vi "FPGA_VI.vi"() -> ()   [LabVIEW 2014]
uses:
  FPGA_Controls/IOClockState.ctl
  <vilib>/Platform/TimedLoop/XDataNode/timing_clust.ctl
  <vilib>/Platform/TimedLoop/XDataNode/nitl_modes.ctl
  <vilib>/Platform/TimedLoop/XDataNode/wakeup.ctl
  FPGA_Controls/DRAMClockState.ctl
  <vilib>/rvi/Emulation/niFpgaSctlEmulationGetInTimedLoop.vi
  <vilib>/rvi/Emulation/niFpgaEmulationReportErrorSimple.vi
  <vilib>/rvi/Emulation/niFpgaGetClockAttributes.vi
  <vilib>/rvi/Emulation/niFpgaCriticalErrorInLSC.vi
  <vilib>/rvi/eio/common/nirviEmuTemplateMethod_errors.vi
  <vilib>/rvi/Emulation/niFpgaEmulationIsFPGAContextNoSignature.vi
  <vilib>/rvi/errors/niFpgaSetErrorForExecOnDevCompSimple.vi
  <vilib>/rvi/eio/common/nirviEmuReportErrorAndStop.vi
  <vilib>/rvi/DataTransferAndStorage/Container/Common/niFpgaContainerGetUniqueNameForEmu.vi
  <vilib>/rvi/FIFO/Fifo_Resource/nirvififoEmulationSetSize.vi
  <vilib>/rvi/FIFO/Fifo_Resource/nirviFifoEmulationQueueMgr.vi
  <instcachedir>/0/nirviFifoEmulationQueueMgr_E5CAEC123FF24DC58D834DCA3CDAA9B5.lvgen/nirviFifoEmulationQueueMgr_E5CAEC123FF24DC58D834DCA3CDAA9B5_002.vi
  <vilib>/Utility/error.llb/Clear Errors.vi
  <vilib>/rvi/FIFO/Fifo_Resource/nirvififoEmulationCreateLock.vi
  <vilib>/rvi/Emulation/niFpgaProcessEmulError.vi
  <vilib>/rvi/FIFO/Fifo_Resource/nirvififoEmulationObtainLock.vi
  <vilib>/rvi/FIFO/Fifo_Resource/nirvififoEmulationReleaseLock.vi
  <vilib>/rvi/occurrence/nirviWaitOnOccurrenceBase.vi
  <vilib>/rvi/errors/nirviReportUnexpectedCaseInternalError.vi
  <vilib>/rvi/errors/nirviReportUnexpectedCaseInternalError (U32).vi
  <vilib>/rvi/interface/RandomDataEmulation/niFpgaRandomDataHandleErrors.vi
  <vilib>/Platform/TimedLoop/XDataNode/XDataNode.xnode
  <vilib>/eio/EIONode/EIONode.xnode
  <vilib>/rvi/DataTransferAndStorage/Container/XNode/niFpgaContainer.xnode
  <vilib>/rvi/FIFO/Fifo_Resource/nirvififoEmulationRead.vi
  <vilib>/rvi/interface/RandomDataEmulation/nirviRandomDataFpgaReadWriteTemplate.vi
  <vilib>/Platform/TimedLoop/XDataNode/XDNodeRunTimeDep.lvlib
panel:
  out "elements written":i32
  out "Init Done":bool
  in  "Trigger":bool
  out "Acquisition \nState":T1
  # "Status"
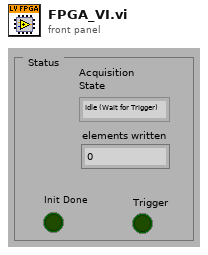
[diagram p1: front panel]
types:
  T1 = typedef "IOClockState.ctl" = enum16{"Idle (Wait for Trigger)", "Aquire"}
  T2 = typedef "XDNodeRunTimeDep.lvlib/timing_clust.ctl" = cluster{"Expected End [f-1]":u64, "Actual End [f-1]":u64, "Finished Late? [f-1]":bool, "Expected End [i-1]":u64, "Actual End [i-1]":u64, "Finished Late? [i-1]":bool, "Expected Start [i]":u64, "Actual Start [i]":u64, "Expected Start [f]":u64, "Actual Start [f]":u64, "Source Name":string, "Structure Name":string, "Period":i64, "Deadline":i64, "Offset":i64, "Start":i64, "Priority":i32, "Timeout":i32, "Mode":T3, "Wakeup Reason":T4, "Error":errorcluster, "Source Type":string, "Secondary Source Type":string, "Global End Time":u64, "Global Start Time":u64, "Frame Duration":u64, "Iteration Duration":u64, "Assigned CPU":i32, "I/O Scan Engine Mode":u32}
  T3 = typedef "XDNodeRunTimeDep.lvlib/nitl_modes.ctl" = enum32{"No Change", "Process missed periods, maintain original phase", "Discard missed periods, maintain original phase", "Process missed periods, ignore original phase", "Discard missed periods, ignore original phase"}
  T4 = typedef "XDNodeRunTimeDep.lvlib/wakeup.ctl" = enum32{"Normal", "Aborted", "Asynchronous wakeup", "Timing source error", "Timed loop error", "Timeout"}
  T5 = typedef "DRAMClockState.ctl" = enum16{"0-7 to DRAM", "8-15 to DRAM", "Read out DRAM 0", "Read out DRAM 1", "Idle"}
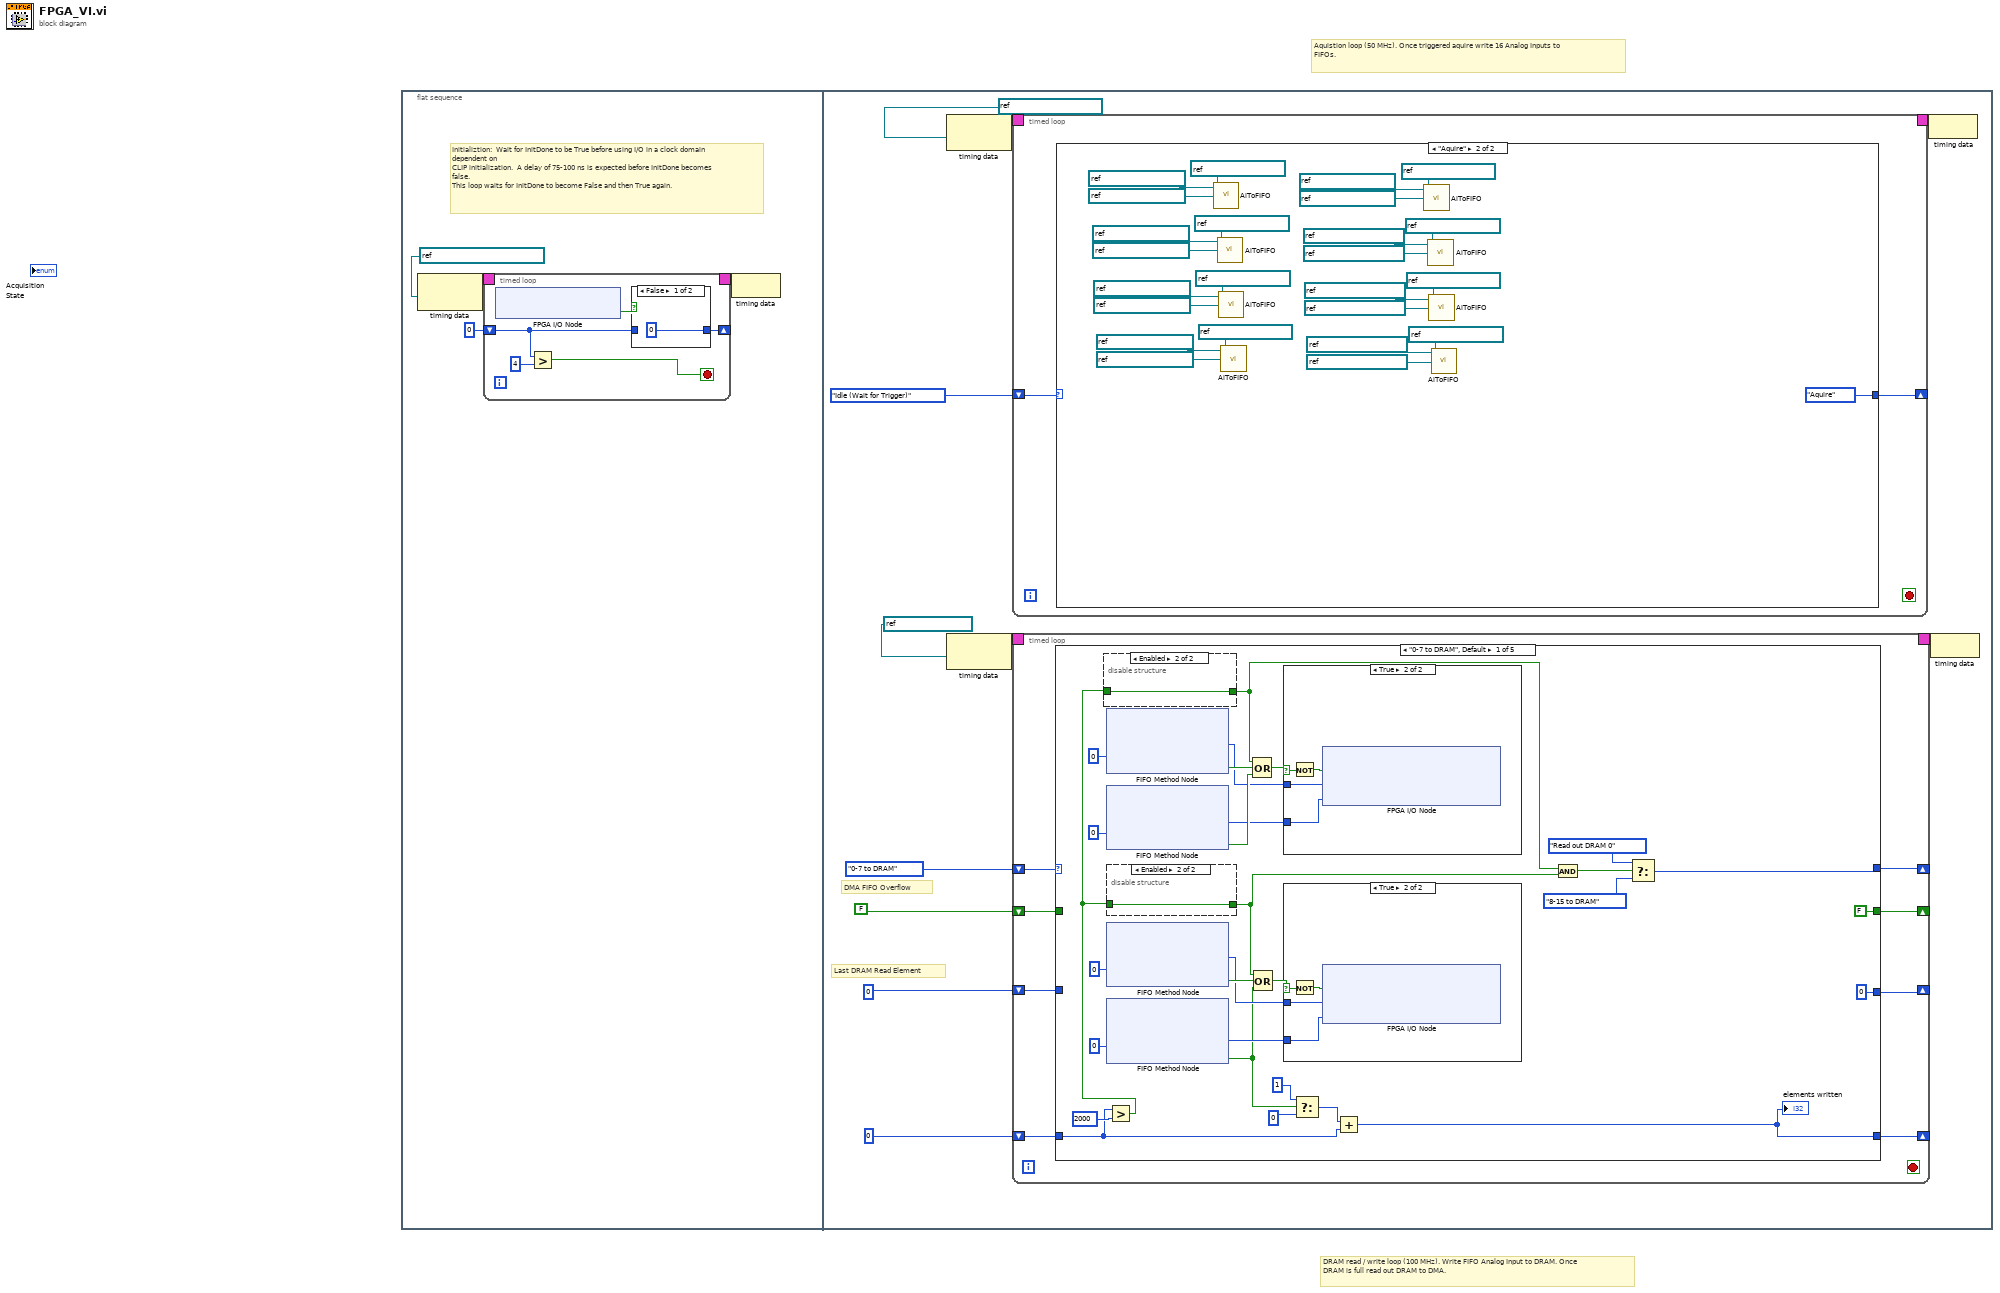
[diagram p0: block diagram]
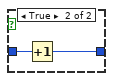
[diagram p2: hidden frame]
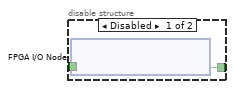
[diagram p3: hidden frame]
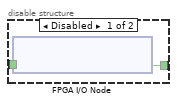
[diagram p4: hidden frame]
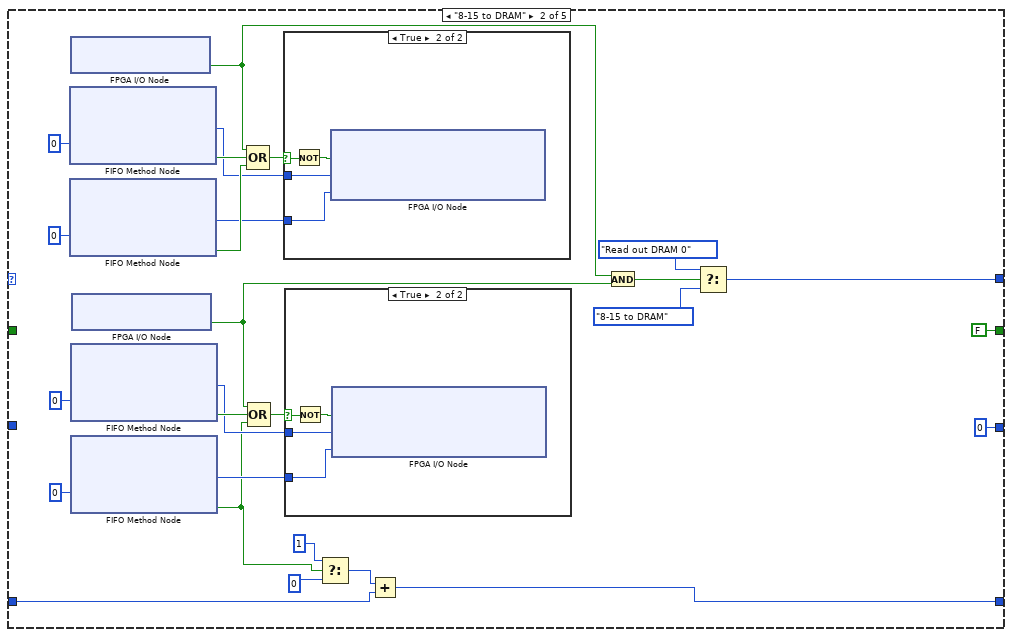
[diagram p7: hidden frame]
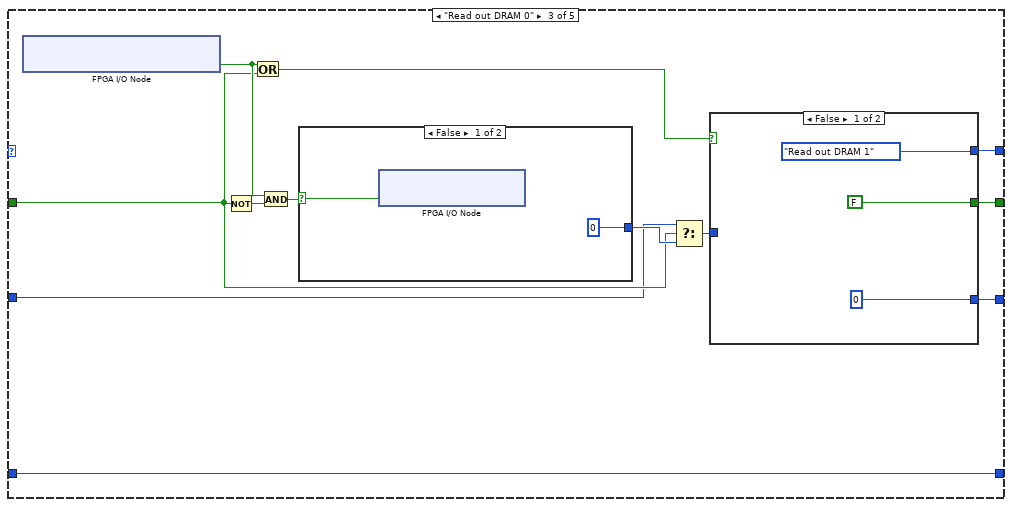
[diagram p10: hidden frame]
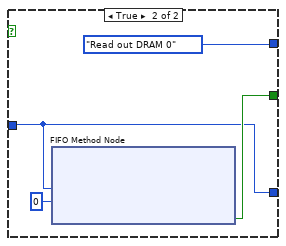
[diagram p11: hidden frame]
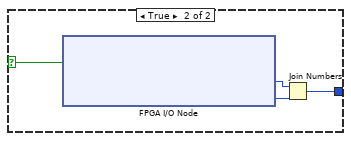
[diagram p12: hidden frame]
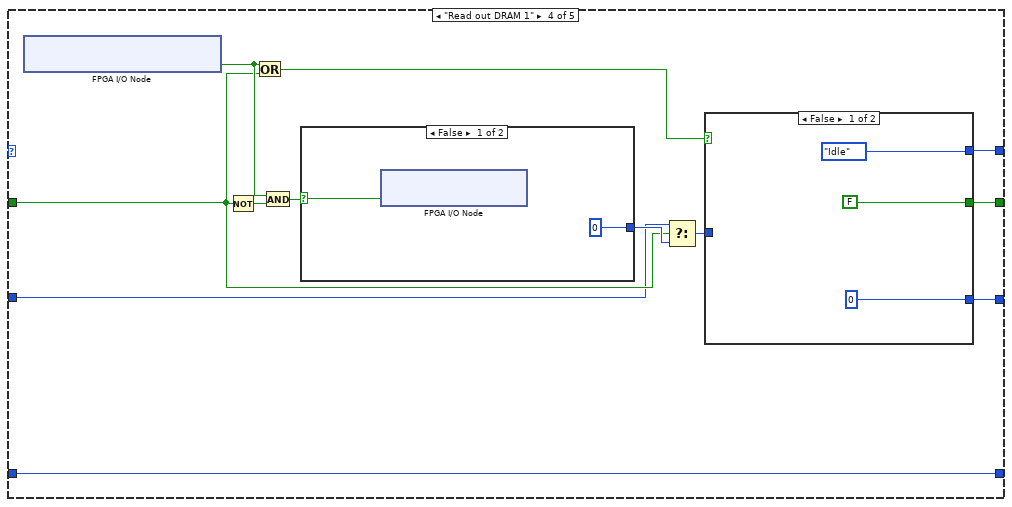
[diagram p13: hidden frame]
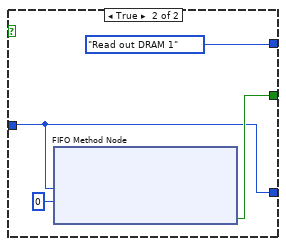
[diagram p14: hidden frame]
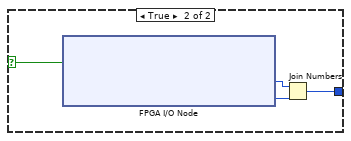
[diagram p15: hidden frame]
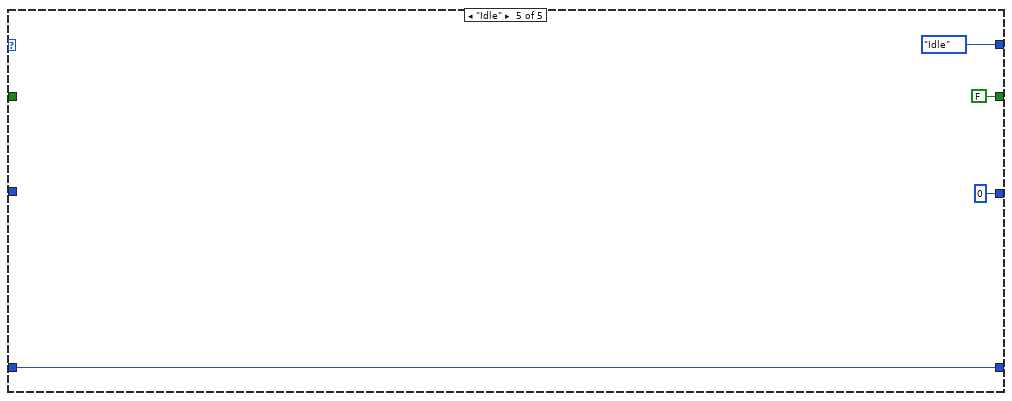
[diagram p16: hidden frame]
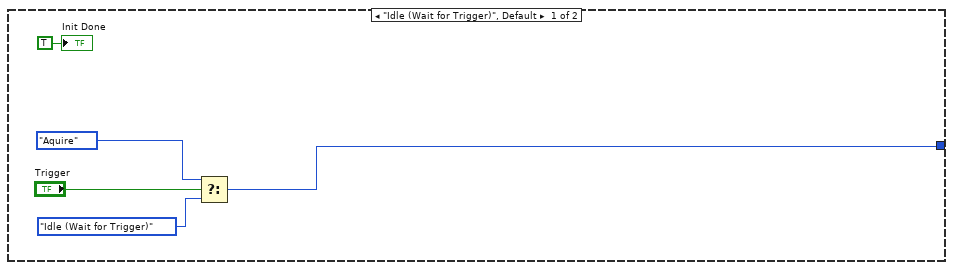
[diagram p17: hidden frame]
diagram:
  # "DRAM read / write loop (100 MHz). Write FIFO Analog Input to DRAM. Once DRAM is full read out DRAM to DMA."
  # "Aquistion loop (50 MHz). Once triggered aquire write 16 Analog Inputs to FIFOs."
  n1 = flat-sequence {
    frame #0 {
      # "Initializtion:  Wait for InitDone to be True before using I/O in a clock domain dependent on \nCLIP initialization.  A delay of 75-100 ns is expected before InitDone becomes false.  \nThis loop waits for InitDone to become False and then True again."
      n2 = node-c288(refnum<k21> "40 MHz Onboard Clock" ("Source Name")) -> (w4:T2)
      n3 = timed-loop {
        shift-right: [w8] -> _
        shift-left: u16 0 -> [w7]
        timing: w4 -> [_]
        timing-out: [_] -> w3
        stop <- w5 stop-if-true
        n4 = xnode "FPGA I/O Node"() -> ("IO Module\\InitDone"=w9:bool)  [unwired: 1 in, 1 out]
        n5 = Greater?(x=w7, y=u16 4) -> (0:w5:bool)
        n6 = case shown="False" w9 {
          tunnel: [u16 0 w12] -> w8
          tunnel: w7 -> [_ w11]
          frame False {
          }
          frame True {
            n7 = Increment(x=w11) -> (x+1=w12:u16)
          }
        }
      }
      n8 = node-c288(w3) -> ()
    }
    frame #1 {
      # "DMA FIFO Overflow"
      # "Last DRAM Read Element"
      n9 = node-c288(refnum<k21> "IO Module Clock 0" ("Source Name")) -> (w29:T2)
      n10 = node-c288(refnum<k21> "100 MHz Clock" ("Source Name")) -> (w26:T2)
      n11 = timed-loop {
        timing: w29 -> [_]
        timing-out: [_] -> w28
        shift-right: [w174] -> _
        shift-left: IOClockState."Idle (Wait for Trigger)" ("AquistionState") -> [w175]
        stop <- _ stop-if-true
        n12 = case shown="\"Aquire\"" w175 {
          tunnel: [w177 IOClockState."Aquire" ("AquistionState")] -> w174
          frame "Idle (Wait for Trigger)", Default {
            n13 = Select(t=IOClockState."Aquire" ("AquistionState"), s="Trigger", f=IOClockState."Idle (Wait for Trigger)" ("AquistionState")) -> (s? t:f=w177:T1)
            "Init Done" <- TRUE ("Init Done")
          }
          frame "Aquire" {
            n14 = call "AiToFIFO.vi"("FIFO"=refnum<k21> "AI-DRAM FIFO 0", "FPGA I/O 1"=refnum<k21> "IO Module\\AI A1" ("FPGA I/O"), "FPGA I/O 0"=refnum<k21> "IO Module\\AI A0" ("FPGA I/O")) -> ()  [unwired: 1 in]
            n15 = call "AiToFIFO.vi"("FIFO"=refnum<k21> "AI-DRAM FIFO 1", "FPGA I/O 1"=refnum<k21> "IO Module\\AI A3" ("FPGA I/O"), "FPGA I/O 0"=refnum<k21> "IO Module\\AI A2" ("FPGA I/O")) -> ()  [unwired: 1 in]
            n16 = call "AiToFIFO.vi"("FIFO"=refnum<k21> "AI-DRAM FIFO 2", "FPGA I/O 1"=refnum<k21> "IO Module\\AI A5" ("FPGA I/O"), "FPGA I/O 0"=refnum<k21> "IO Module\\AI A4" ("FPGA I/O")) -> ()  [unwired: 1 in]
            n17 = call "AiToFIFO.vi"("FIFO"=refnum<k21> "AI-DRAM FIFO 3", "FPGA I/O 1"=refnum<k21> "IO Module\\AI A7" ("FPGA I/O"), "FPGA I/O 0"=refnum<k21> "IO Module\\AI A6" ("FPGA I/O")) -> ()  [unwired: 1 in]
            n18 = call "AiToFIFO.vi"("FIFO"=refnum<k21> "AI-DRAM FIFO 4", "FPGA I/O 1"=refnum<k21> "IO Module\\AI B9" ("FPGA I/O"), "FPGA I/O 0"=refnum<k21> "IO Module\\AI B8" ("FPGA I/O")) -> ()  [unwired: 1 in]
            n19 = call "AiToFIFO.vi"("FIFO"=refnum<k21> "AI-DRAM FIFO 5", "FPGA I/O 1"=refnum<k21> "IO Module\\AI B11" ("FPGA I/O"), "FPGA I/O 0"=refnum<k21> "IO Module\\AI B10" ("FPGA I/O")) -> ()  [unwired: 1 in]
            n20 = call "AiToFIFO.vi"("FIFO"=refnum<k21> "AI-DRAM FIFO 6", "FPGA I/O 1"=refnum<k21> "IO Module\\AI B13" ("FPGA I/O"), "FPGA I/O 0"=refnum<k21> "IO Module\\AI B12" ("FPGA I/O")) -> ()  [unwired: 1 in]
            n21 = call "AiToFIFO.vi"("FIFO"=refnum<k21> "AI-DRAM FIFO 7", "FPGA I/O 1"=refnum<k21> "IO Module\\AI B15" ("FPGA I/O"), "FPGA I/O 0"=refnum<k21> "IO Module\\AI B14" ("FPGA I/O")) -> ()  [unwired: 1 in]
          }
        }
      }
      n22 = timed-loop {
        timing: w26 -> [_]
        timing-out: [_] -> w25
        shift-right: [w34] -> _
        shift-left: FALSE ("Timed Out?") -> [w37]
        shift-right: [w35] -> _
        shift-left: u64 0 ("Timeout") -> [w36]
        shift-right: [w32] -> _
        shift-left: DRAMClockState."0-7 to DRAM" -> [w33]
        shift-right: [w30] -> _
        shift-left: 0 -> [w31]
        stop <- _ stop-if-true
        n23 = case shown="\"0-7 to DRAM\", Default" w33 {
          tunnel: w37 -> [_ _ w119 w144 _]
          tunnel: w36 -> [_ _ w118 w143 _]
          tunnel: [u64 0 ("Timeout") u64 0 ("Timeout") w117 w142 u64 0 ("Timeout")] -> w35
          tunnel: [FALSE ("Timed Out?") FALSE ("Timed Out?") w116 w141 FALSE ("Timed Out?")] -> w34
          tunnel: [w46 w85 w115 w140 DRAMClockState."Idle"] -> w32
          tunnel: w31 -> [w38 w80 w114 w139 w164]
          tunnel: [w41 w79 w114 w139 w164] -> w30
          frame "0-7 to DRAM", Default {
            n24 = xnode ("FIFO Method Node")("Timeout"=0) -> ("Element"=w63:u32, "Timed Out?"=w64:bool)  [unwired: 1 in, 1 out]
            n25 = xnode ("FIFO Method Node")("Timeout"=0) -> ("Element"=w62:u32, "Timed Out?"=w65:bool)  [unwired: 1 in, 1 out]
            n26 = xnode ("FIFO Method Node")("Timeout"=0) -> ("Element"=w59:u32, "Timed Out?"=w60:bool)  [unwired: 1 in, 1 out]
            n27 = xnode ("FIFO Method Node")("Timeout"=0) -> ("Element"=w58:u32, "Timed Out?"=w45:bool)  [unwired: 1 in, 1 out]
            n28 = Greater?(x=w38, y=2000 ("x")) -> (0:w40:bool)
            n29 = disable-structure shown="Enabled" {
              disable-tunnel: [w69 w70] -> w52
              disable-tunnel: w40 -> [_ w70]
              frame Disabled {
                n30 = xnode "FPGA I/O Node"() -> ("DRAM Bank 0\\Full"=w69:bool)  [unwired: 1 in, 1 out]
              }
              frame Enabled {
              }
            }
            n31 = disable-structure shown="Enabled" {
              disable-tunnel: [w67 w68] -> w53
              disable-tunnel: w40 -> [_ w68]
              frame Disabled {
                n32 = xnode "FPGA I/O Node"() -> ("DRAM Bank 1\\Full"=w67:bool)  [unwired: 1 in, 1 out]
              }
              frame Enabled {
              }
            }
            n33 = Compound Arithmetic op=OR(w52, w64, w65) -> (w66:bool)
            n34 = Compound Arithmetic op=OR(w53, w60, w45) -> (w61:bool)
            n35 = case shown="True" w66 {
              selector: w66 -> [_ w78]
              tunnel: w63 -> [_ w76]
              tunnel: w62 -> [_ w75]
              frame False {
              }
              frame True {
                n36 = Not(x=w78) -> (.not. x?=w77:bool)
                n37 = xnode "FPGA I/O Node"("DRAM Bank 0\\Write"=w77, "DRAM Bank 0\\Write_Data_Upper"=w76, "DRAM Bank 0\\Write_Data_Lower"=w75) -> ()  [unwired: 3 in, 3 out]
              }
            }
            n38 = case shown="True" w61 {
              selector: w61 -> [_ w74]
              tunnel: w59 -> [_ w72]
              tunnel: w58 -> [_ w71]
              frame False {
              }
              frame True {
                n39 = Not(x=w74) -> (.not. x?=w73:bool)
                n40 = xnode "FPGA I/O Node"("DRAM Bank 1\\Write"=w73, "DRAM Bank 1\\Write_Data_Upper"=w72, "DRAM Bank 1\\Write_Data_Lower"=w71) -> ()  [unwired: 3 in, 3 out]
              }
            }
            n41 = Select(t=1, s=w45, f=0) -> (s? t:f=w42:i32)
            n42 = Add(x=w42, y=w38) -> (x+y=w41:i32)
            "elements written" <- w41
            n43 = And(x=w52, y=w53) -> (x .and. y?=w51:bool)
            n44 = Select(t=DRAMClockState."Read out DRAM 0", s=w51, f=DRAMClockState."8-15 to DRAM") -> (s? t:f=w46:T5)
          }
          frame "8-15 to DRAM" {
            n45 = xnode ("FIFO Method Node")("Timeout"=0) -> ("Element"=w102:u32, "Timed Out?"=w103:bool)  [unwired: 1 in, 1 out]
            n46 = xnode ("FIFO Method Node")("Timeout"=0) -> ("Element"=w101:u32, "Timed Out?"=w104:bool)  [unwired: 1 in, 1 out]
            n47 = xnode "FPGA I/O Node"() -> ("DRAM Bank 0\\Full"=w89:bool)  [unwired: 1 in, 1 out]
            n48 = xnode ("FIFO Method Node")("Timeout"=0) -> ("Element"=w98:u32, "Timed Out?"=w99:bool)  [unwired: 1 in, 1 out]
            n49 = xnode ("FIFO Method Node")("Timeout"=0) -> ("Element"=w97:u32, "Timed Out?"=w81:bool)  [unwired: 1 in, 1 out]
            n50 = xnode "FPGA I/O Node"() -> ("DRAM Bank 1\\Full"=w88:bool)  [unwired: 1 in, 1 out]
            n51 = Compound Arithmetic op=OR(w89, w103, w104) -> (w105:bool)
            n52 = Compound Arithmetic op=OR(w88, w99, w81) -> (w100:bool)
            n53 = case shown="True" w105 {
              selector: w105 -> [_ w113]
              tunnel: w102 -> [_ w111]
              tunnel: w101 -> [_ w110]
              frame False {
              }
              frame True {
                n54 = Not(x=w113) -> (.not. x?=w112:bool)
                n55 = xnode "FPGA I/O Node"("DRAM Bank 0\\Write"=w112, "DRAM Bank 0\\Write_Data_Upper"=w111, "DRAM Bank 0\\Write_Data_Lower"=w110) -> ()  [unwired: 3 in, 3 out]
              }
            }
            n56 = case shown="True" w100 {
              selector: w100 -> [_ w109]
              tunnel: w98 -> [_ w107]
              tunnel: w97 -> [_ w106]
              frame False {
              }
              frame True {
                n57 = Not(x=w109) -> (.not. x?=w108:bool)
                n58 = xnode "FPGA I/O Node"("DRAM Bank 1\\Write"=w108, "DRAM Bank 1\\Write_Data_Upper"=w107, "DRAM Bank 1\\Write_Data_Lower"=w106) -> ()  [unwired: 3 in, 3 out]
              }
            }
            n59 = Select(t=1, s=w81, f=0) -> (s? t:f=w82:i32)
            n60 = Add(x=w82, y=w80) -> (x+y=w79:i32)
            n61 = And(x=w89, y=w88) -> (x .and. y?=w92:bool)
            n62 = Select(t=DRAMClockState."Read out DRAM 0", s=w92, f=DRAMClockState."8-15 to DRAM") -> (s? t:f=w85:T5)
          }
          frame "Read out DRAM 0" {
            n63 = xnode "FPGA I/O Node"() -> ("DRAM Bank 0\\Data_Available"=w122:bool)  [unwired: 1 in, 1 out]
            n64 = Not(x=w119) -> (.not. x?=w121:bool)
            n65 = Or(x=w122, y=w119) -> (x .or. y?=w125:bool)
            n66 = And(x=w122, y=w121) -> (x .and. y?=w120:bool)
            n67 = case shown="False" w120 {
              selector: w120 -> [w133 w136]
              tunnel: [u64 0 ("Timeout") w135] -> w123
              frame False {
                n68 = xnode "FPGA I/O Node"("DRAM Bank 0\\Read"=w133) -> ()  [unwired: 1 in, 1 out]
              }
              frame True {
                n69 = xnode "FPGA I/O Node"("DRAM Bank 0\\Read"=w136) -> ("DRAM Bank 0\\Read_Data_Upper"=w137:u32, "DRAM Bank 0\\Read_Data_Lower"=w138:u32)  [unwired: 3 in, 3 out]
                n70 = Join Numbers(hi=w137, lo=w138) -> ((hi.lo)=w135:u64)
              }
            }
            n71 = Select(t=w118, s=w119, f=w123) -> (s? t:f=w124:u64)
            n72 = case shown="False" w125 {
              tunnel: [DRAMClockState."Read out DRAM 1" DRAMClockState."Read out DRAM 0"] -> w115
              tunnel: w124 -> [_ w129]
              tunnel: [u64 0 ("Timeout") w129] -> w117
              tunnel: [FALSE ("Timed Out?") w130] -> w116
              frame False {
              }
              frame True {
                n73 = xnode ("FIFO Method Node")("Element"=w129, "Timeout"=0) -> ("Timed Out?"=w130:bool)  [unwired: 1 in, 1 out]
              }
            }
          }
          frame "Read out DRAM 1" {
            n74 = xnode "FPGA I/O Node"() -> ("DRAM Bank 1\\Data_Available"=w147:bool)  [unwired: 1 in, 1 out]
            n75 = Not(x=w144) -> (.not. x?=w146:bool)
            n76 = Or(x=w147, y=w144) -> (x .or. y?=w150:bool)
            n77 = And(x=w147, y=w146) -> (x .and. y?=w145:bool)
            n78 = case shown="False" w145 {
              selector: w145 -> [w158 w161]
              tunnel: [u64 0 ("Timeout") w160] -> w148
              frame False {
                n79 = xnode "FPGA I/O Node"("DRAM Bank 1\\Read"=w158) -> ()  [unwired: 1 in, 1 out]
              }
              frame True {
                n80 = xnode "FPGA I/O Node"("DRAM Bank 1\\Read"=w161) -> ("DRAM Bank 1\\Read_Data_Upper"=w162:u32, "DRAM Bank 1\\Read_Data_Lower"=w163:u32)  [unwired: 3 in, 3 out]
                n81 = Join Numbers(hi=w162, lo=w163) -> ((hi.lo)=w160:u64)
              }
            }
            n82 = Select(t=w143, s=w144, f=w148) -> (s? t:f=w149:u64)
            n83 = case shown="False" w150 {
              tunnel: [DRAMClockState."Idle" DRAMClockState."Read out DRAM 1"] -> w140
              tunnel: w149 -> [_ w154]
              tunnel: [u64 0 ("Timeout") w154] -> w142
              tunnel: [FALSE ("Timed Out?") w155] -> w141
              frame False {
              }
              frame True {
                n84 = xnode ("FIFO Method Node")("Element"=w154, "Timeout"=0) -> ("Timed Out?"=w155:bool)  [unwired: 1 in, 1 out]
              }
            }
          }
          frame "Idle" {
          }
        }
      }
      n85 = node-c288(w28) -> ()
      n86 = node-c288(w25) -> ()
    }
  }
